vi "Circulo.vi"() -> ()   [LabVIEW 2020]
panel:
  out "Gráfico de un circulo":cluster{dbl[], dbl[]}(graph)
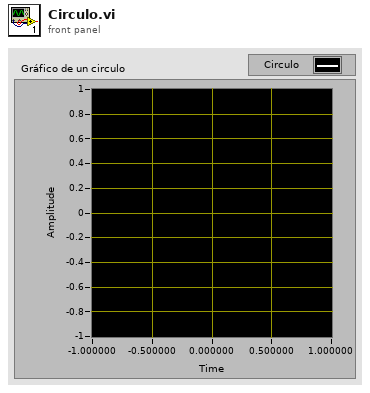
[diagram p1: front panel]
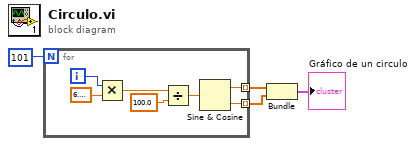
[diagram p0: block diagram]
diagram:
  n1 = for {
    N: 101 -> [_]
    tunnel: [w7] -> w3 mode=indexing
    tunnel: [w6] -> w2 mode=indexing
    i -> [w11]
    n2 = Multiply(x=w11, y=6.283185307179586) -> (x*y=w10:dbl)
    n3 = Divide(x=w10, y=100.0) -> (x/y=w8:dbl)
    n4 = Sine & Cosine(0:w8) -> (1:w7:dbl, 2:w6:dbl)
  }
  n5 = Bundle(w3, w2) -> (→"Gráfico de un circulo":cluster{dbl[], dbl[]})  [unwired: 1 in]
